vi "14 Saving and Reading Files.vi"() -> ()   [LabVIEW 2019]
uses:
  _Subs/OpenDiagram/Open_XControl.xctl
  <vilib>/Utility/file.llb/Write Delimited Spreadsheet (DBL).vi
  <vilib>/Utility/file.llb/Read Delimited Spreadsheet (DBL).vi
panel:
  out "txt files in your temp folder":string[](array[string])
  out "Numbers read":dbl[](array[numeric])
  in  "Numbers to save":dbl[](array[numeric])
  out "Text read":string
  in  "Path to file":path
  in  "OpenDiag":refnum<vi>(xcontrol)
  # "14 Saving and Reading Files\nThis code will save and then read a text file\n\nInstructions:\n1. Click on the folder icon to create your new file path and file name\n2. Hit the Run arrow and see the code execute"
  # "WRITE THEN READ FILE"
  # "READ FROM FILE"
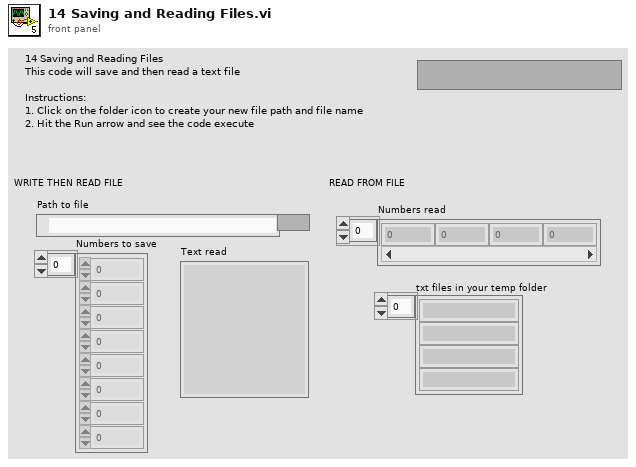
[diagram p1: front panel]
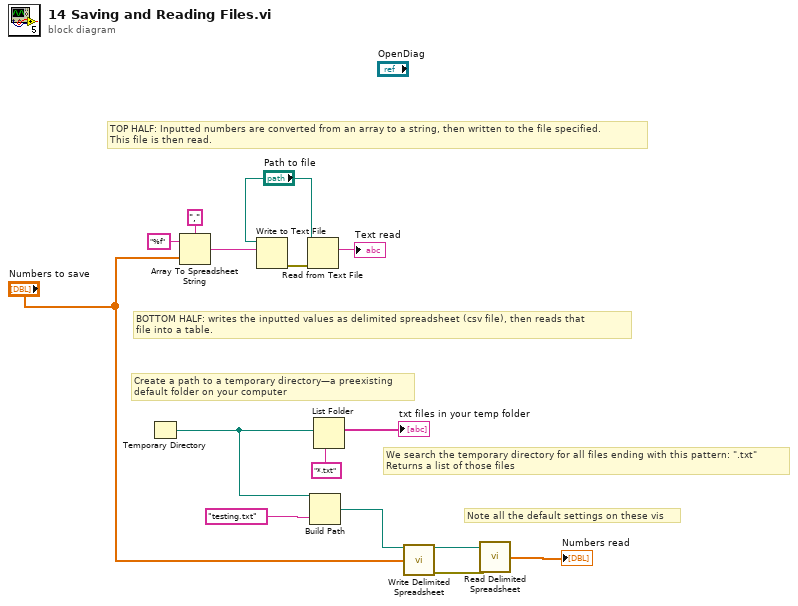
[diagram p0: block diagram]
diagram:
  # "We search the temporary directory for all files ending with this pattern: \".txt\"\nReturns a list of those files"
  # "Create a path to a temporary directory—a preexisting\ndefault folder on your computer"
  # "BOTTOM HALF: writes the inputted values as delimited spreadsheet (csv file), then reads that \nfile into a table."
  # "TOP HALF: Inputted numbers are converted from an array to a string, then written to the file specified.\nThis file is then read."
  # "Note all the default settings on these vis"
  n1 = Temporary Directory() -> (w4:path)
  n2 = Array To Spreadsheet String(delimiter (Tab)=",", array="Numbers to save", 3:"%f" ("format string")) -> (spreadsheet string=w10:string)
  n3 = Write to Text File(file (use dialog)="Path to file", text=w10) -> (error out=w15:errorcluster)  [unwired: 2 in, 2 out]
  n4 = Read from Text File(file (use dialog)="Path to file", error in=w15) -> (text=→"Text read":string)  [unwired: 2 in, 3 out]
  n5 = Build Path(base path=w4, name or relative path="testing.txt") -> (appended path=w1:path)
  n6 = List Folder(path=w4, pattern="*.txt") -> (filenames=→"txt files in your temp folder":string[])  [unwired: 2 in, 3 out]
  n7 = call-poly <vilib>:"Write Delimited Spreadsheet.vi"("file path (dialog if empty)"=w1, "1D data"="Numbers to save") -> ("new file path (Not A Path if cancelled)"=w8:path, "error out"=w7:errorcluster)  [unwired: 12 in]
  n8 = call-poly <vilib>:"Read Delimited Spreadsheet.vi"("file path (dialog if empty)"=w8, "error in (no error)"=w7) -> ("first row"=→"Numbers read":dbl[])  [unwired: 8 in, 5 out]
